vi "Read.vi"(11 "StatusTreeValue in":refnum<class "StatusTreeValue.lvclass">) -> (2 "Status Tree":map{string[], T1}(c390))   [LabVIEW 2020, in "Volatus.lvlib" / "StatusTreeValue.lvclass"]
uses:
  StatusTreeValue.lvclass
  StatusTreeValue.lvclass/StatusTreeValue.ctl
  Module/State.ctl
  Module/Module.lvclass
  Module Status.ctl
  Volatus.lvlib
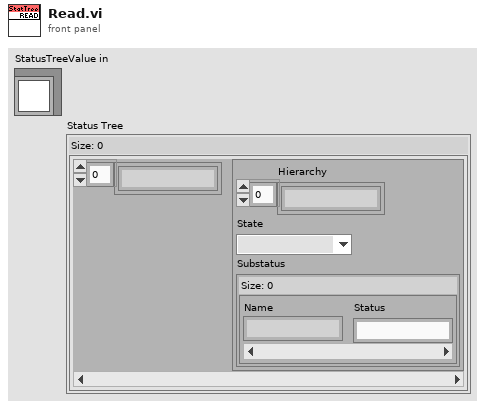
[diagram p1: front panel]
types:
  T1 = typedef "Volatus.lvlib/Module Status.ctl" = cluster{"Hierarchy":string[], "State":T2, "Substatus":map{string, string}}
  T2 = typedef "Volatus.lvlib/Module.lvclass/State.ctl" = enum16{"Unknown", "Launched", "Starting", "Running", "Stopping", "Stopped", "Error - Starting", "Error - Run", "Error - Stopping"}
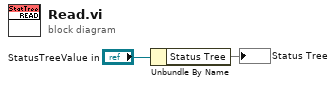
[diagram p0: block diagram]
diagram:
  n1 = Unbundle By Name("StatusTreeValue in") -> ("Status Tree"=→"Status Tree":map{string[], T1})
